vi "Get I32.vi"(8 "error in (no error)":errorcluster, 9 "Data Type (default value)":i32, 10 "Offset":i32, 11 "JSON":string) -> (0 "error out":errorcluster, 1 "Number":i32)   [LabVIEW 2015, in "JSONtext.lvlib"]
uses:
  JSONtext.lvlib
  String Subset.vi
  Advance past Number.vi
  Parsing Error.vi
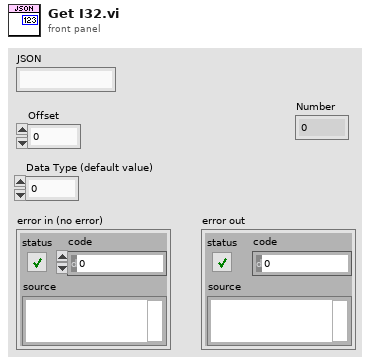
[diagram p1: front panel]
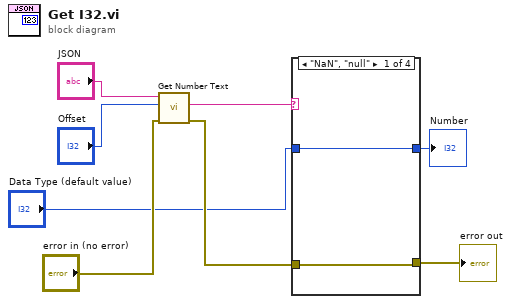
[diagram p0: block diagram]
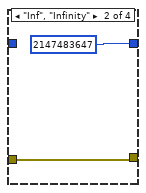
[diagram p2: hidden frame]
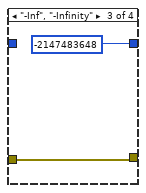
[diagram p3: hidden frame]
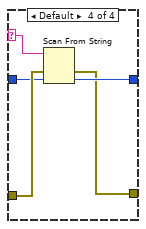
[diagram p4: hidden frame]
diagram:
  n1 = call "Get Number Text.vi"("error in (no error)"="error in (no error)", "Offset"="Offset", "JSON"="JSON") -> ("error out"=w5:errorcluster, "Number Text"=w3:string)  [unwired: 6 in, 1 out]
  n2 = case shown="\"NaN\", \"null\"" w3 {
    selector: w3 -> [_ _ _ w15]
    tunnel: [w9 2147483647 ("default value 1") -2147483648 ("default value 1") w19] -> w2
    tunnel: w5 -> [w10 w11 w13 w18]
    tunnel: [w10 w11 w13 w17] -> w4
    tunnel: "Data Type (default value)" -> [w9 _ _ w16]
    frame "NaN", "null" {
    }
    frame "Inf", "Infinity" {
    }
    frame "-Inf", "-Infinity" {
    }
    frame Default {
      n3 = Scan From String(input string=w15, error in=w18, default 1=w16) -> (error out=w17:errorcluster, output 1=w19:i32)  [unwired: 2 in, 2 out]
    }
  }
  "error out" <- w4
  "Number" <- w2
